vi "DeleteProxyObject.vi"(1 "remote object ref":refnum<class "G#Object.lvclass">, 5 "error in (no error)":errorcluster, 6 "force delete? (F)":bool) -> (19 "error out":errorcluster)   [LabVIEW 2017, in "G#RemoteProxy.lvclass"]
doc: "Deletes the proxy object."
uses:
  G#RemoteProxy.lvclass
  G#Object/G#Object.lvclass
  C:/Program Files (x86)/National Instruments/LabVIEW 2017/vi.lib/addons/_AddQ/G#Object/G#Object.lvclass
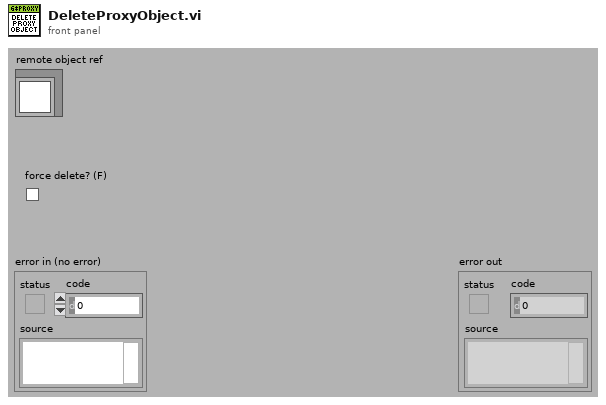
[diagram p1: front panel]
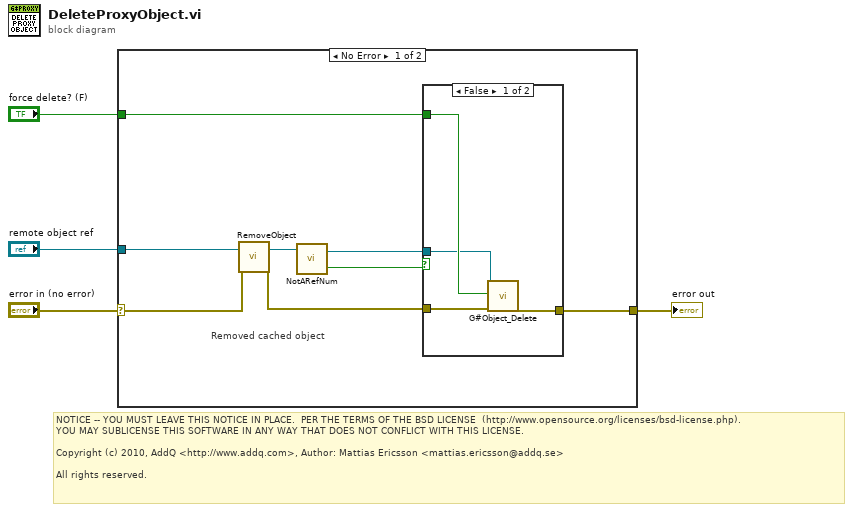
[diagram p0: block diagram]
diagram:
  # "NOTICE -- YOU MUST LEAVE THIS NOTICE IN PLACE.  PER THE TERMS OF THE BSD LICENSE  (http://www.opensource.org/licenses/bsd-license.php).\nYOU MAY SUBLICENSE THIS SOFTWARE IN ANY WAY THAT DOES NOT CONFLICT WITH THIS LICENSE.\n\nCopyright (c) 2010, AddQ <http://www.addq.com>, Author: Mattias Ericsson <mattias.ericsson@addq.se>\n\nAll rights reserved."
  n1 = case shown="No Error" "error in (no error)" {
    selector: "error in (no error)" -> [w10 w18]
    tunnel: [w11 w18] -> w3
    tunnel: "force delete? (F)" -> [w12 _]
    tunnel: "remote object ref" -> [w8 _]
    frame No Error {
      # "Removed cached object"
      n2 = call "RemoveObject.vi"("remote ref"=w8, "error in (no error)"=w10) -> ("proxy ref"=w7:refnum<class "G#RemoteProxy.lvclass">, "error out"=w9:errorcluster)  [unwired: 16 in]
      n3 = call-dynamic "NotARefNum.vi"("reference in"=w7) -> ("not a refnum?"=w5:bool, "reference out"=w6:refnum<class "G#RemoteProxy.lvclass">)  [unwired: 1 in]
      n4 = case shown="False" w5 {
        tunnel: w12 -> [w16 _]
        tunnel: [w15 w17] -> w11
        tunnel: w9 -> [w14 w17]
        tunnel: w6 -> [w13 _]
        frame False {
          n5 = call "G#Object_Delete.vi"("reference in"=w13, "force delete? (F)"=w16, "error in (no error)"=w14) -> ("error out"=w15:errorcluster)  [unwired: 15 in, 1 out]
        }
        frame True {
        }
      }
    }
    frame Error {
    }
  }
  "error out" <- w3
